vi "Disable Message Logging.vi"(8 "error in (no error)":errorcluster, 11 "Monitored Actor in":refnum<class "Monitored Actor.lvclass">) -> (0 "error out":errorcluster, 3 "Monitored Actor out":refnum<class "Monitored Actor.lvclass">)   [LabVIEW 2023, in "Monitored Actor.lvlib" / "Monitored Actor.lvclass"]
doc: "Stops message logging\n\nCopyright: MGI 2016\nAuthor: Derek Trepanier"
uses:
  Monitored Actor.lvclass
  Monitored Actor.lvclass/Monitored Actor.ctl
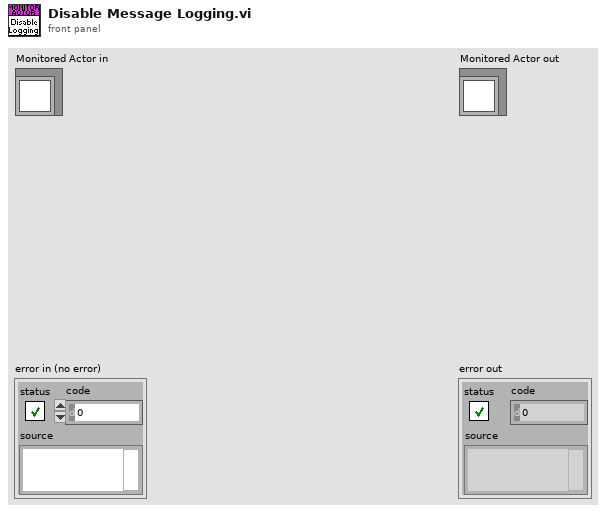
[diagram p1: front panel]
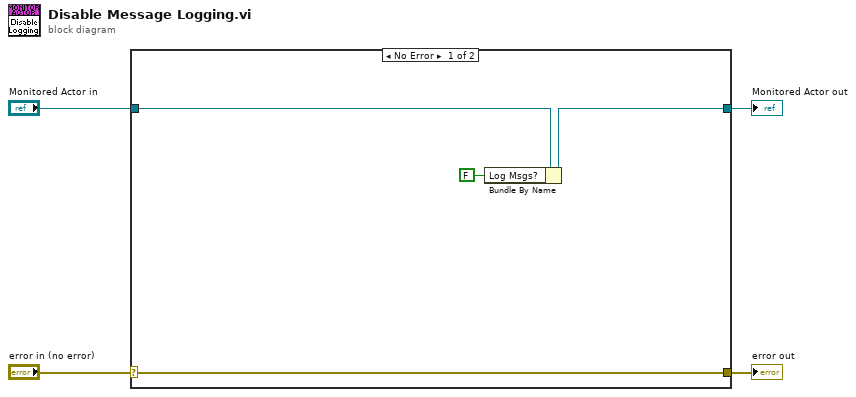
[diagram p0: block diagram]
diagram:
  n1 = case shown="No Error" "error in (no error)" {
    selector: "error in (no error)" -> [w8 w10]
    tunnel: [w8 w10] -> w3
    tunnel: [w6 w9] -> w1
    tunnel: "Monitored Actor in" -> [w7 w9]
    frame No Error {
      n2 = Bundle By Name(cluster=w7, "Log Msgs?"=FALSE) -> (w6:refnum<class "Monitored Actor.lvclass">)
    }
    frame Error {
    }
  }
  "error out" <- w3
  "Monitored Actor out" <- w1
